vi "Get RAG Python Script.vi"(11 "Python RAG Script in":path caption="Embedding Model URL in") -> (3 "Python RAG Script out":path)   [LabVIEW 2023, in "LabVIEW RAG.lvlib"]
uses:
  LabVIEW RAG.lvlib
  AI RAG Globals.vi
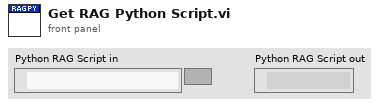
[diagram p1: front panel]
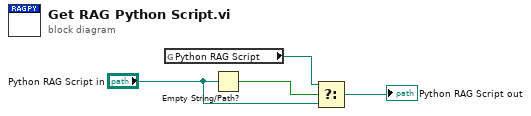
[diagram p0: block diagram]
diagram:
  n1 = global read "AI RAG Globals.vi" "Python RAG Script"() -> (w4:path)
  n2 = Empty String/Path?(string/path="Python RAG Script in") -> (empty?=w3:bool)
  n3 = Select(t=w4, s=w3, f="Python RAG Script in") -> (s? t:f=→"Python RAG Script out":path)
